vi "Fault Handling.vi"(8 "error in (no error)":errorcluster, 10 "FaultCode":i32, 11 "PreUUT in":refnum<class "PreUUT.lvclass">) -> (0 "error out":errorcluster, 3 "PreUUT out":refnum<class "PreUUT.lvclass">)   [LabVIEW 2021, in "PreUUT.lvclass"]
uses:
  PreUUT.lvclass
  PreUUT.lvclass/PreUUT.ctl
  OPC UA/OPC UA.lvclass
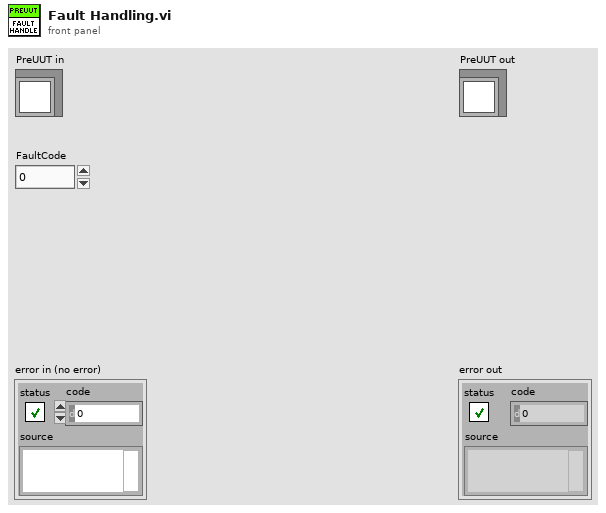
[diagram p1: front panel]
types:
  T1 = typedef "PreUUT.lvclass/Rx PreUUT.ctl" = cluster{"NestStatus":bool, "PalletID":u32, "Start":bool, "BarcodeData":string, "FaultCode":u32, "Stop":bool}
  T2 = typedef "PreUUT.lvclass/Tx PreUUT.ctl" = cluster{"Online":bool, "Ready":bool, "Fault":bool, "Timeout":bool, "Results":u32, "StepNo":u32, "TestRunning":bool, "ResultsReady":bool}
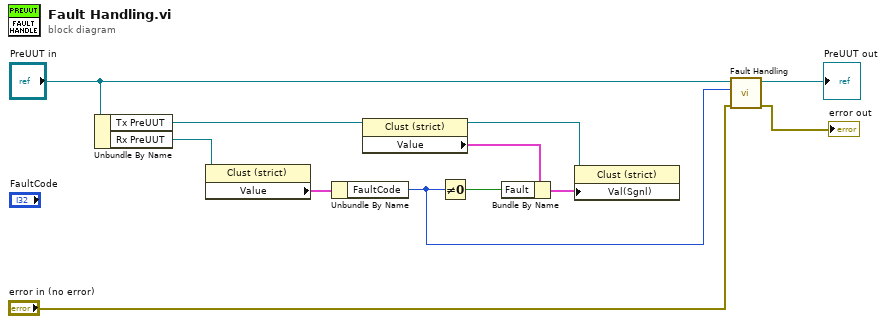
[diagram p0: block diagram]
diagram:
  n1 = Unbundle By Name("PreUUT in") -> ("Tx PreUUT"=w8:refnum<vi>, "Rx PreUUT"=w11:refnum<vi>)
  n2 = property class="Clust (strict)"(reference=w11) -> ("Value"=w10:T1)  [unwired: 1 in, 2 out]
  n3 = Unbundle By Name(w10) -> ("FaultCode"=w3:u32)
  n4 = property class="Clust (strict)"(reference=w8) -> (reference out=w6:refnum<vi>, "Value"=w4:T2)  [unwired: 1 in, 1 out]
  n5 = Not Equal To 0?(x=w3) -> (x != 0?=w1:bool)
  n6 = Bundle By Name(cluster=w4, "Fault"=w1) -> (w7:T2)
  n7 = property class="Clust (strict)"(reference=w6, "Val(Sgnl)"=w7) -> ()  [unwired: 1 in, 2 out]
  n8 = call-parent "Fault Handling.vi"("error in (no error)"="error in (no error)", "FaultCode"=w3, "OPC UA in"="PreUUT in") -> ("error out"=→"error out":errorcluster, "OPC UA out"=→"PreUUT out":refnum<class "PreUUT.lvclass">)  [unwired: 7 in]
